vi "stage_get_current_xyz.vi"(2 "error in":errorcluster) -> (0 "error out":errorcluster, 1 "Aktuelle xyz-Position OUT [mm]":dbl[](array[numeric]))   [LabVIEW 2009]
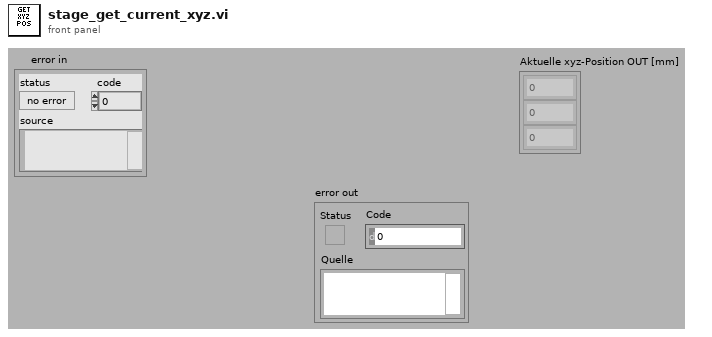
[diagram p1: front panel]
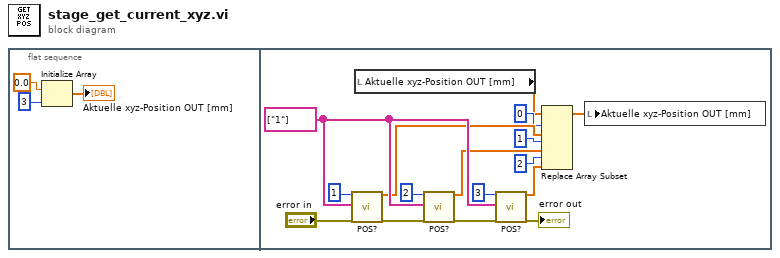
[diagram p0: block diagram]
diagram:
  n1 = flat-sequence {
    frame #0 {
      n2 = Initialize Array(0.0 ("Element"), 3 ("Dimension")) -> (→"Aktuelle xyz-Position OUT [mm]":dbl[])
    }
    frame #1 {
      w19 = string[] ["1"] ("Axes to query")
      n3 = call "POS?.vi"("System no."=1, "Axes to query"=w19, "error in"="error in") -> ("Position"=w13:dbl[], "error out"=w7:errorcluster)  [unwired: 15 in]
      n4 = local read "Aktuelle xyz-Position OUT [mm]"() -> (w6:dbl[])
      n5 = call "POS?.vi"("System no."=2, "Axes to query"=w19, "error in"=w7) -> ("Position"=w14:dbl[], "error out"=w8:errorcluster)  [unwired: 15 in]
      n6 = call "POS?.vi"("System no."=3, "Axes to query"=w19, "error in"=w8) -> ("Position"=w15:dbl[], "error out"=→"error out":errorcluster)  [unwired: 15 in]
      n7 = Replace Array Subset(array=w6, new element #1=w13, index #1=0 ("Index"), new element #2=w14, index #2=1 ("Index"), new element #3=w15, index #3=2 ("Index")) -> (w5:dbl[])
      n8 = local write "Aktuelle xyz-Position OUT [mm]"(w5) -> ()
    }
  }
